vi "Get or Add TableDefinitionPart.vi"(7 "Sheet Name":string, 8 "error in":errorcluster, 10 "Table Name":string, 11 "SpreadsheetDoc in":refnum<k24>) -> (0 "error out":errorcluster, 2 "TableDefinitionPart":refnum<k24>, 3 "SpreadsheetDo out":refnum<k24>, 5 "Sheet Name":string)   [LabVIEW 2019, in "Open Xml.lvlib"]
uses:
  Open Xml.lvlib
  D:/git/Open-Xml-LabVIEW/Source/OpenXmlGenericsWrapper.dll
  OpenXmlGenericsWrapper.dll
  D:/git/Open-Xml-LabVIEW/Source/DocumentFormat.OpenXml.dll
  DocumentFormat.OpenXml.dll
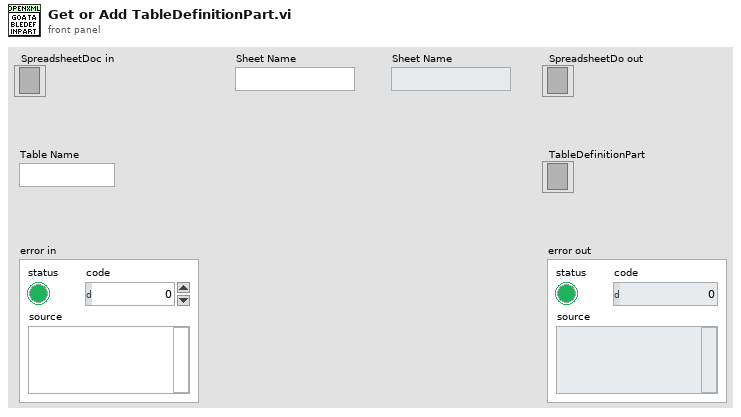
[diagram p1: front panel]
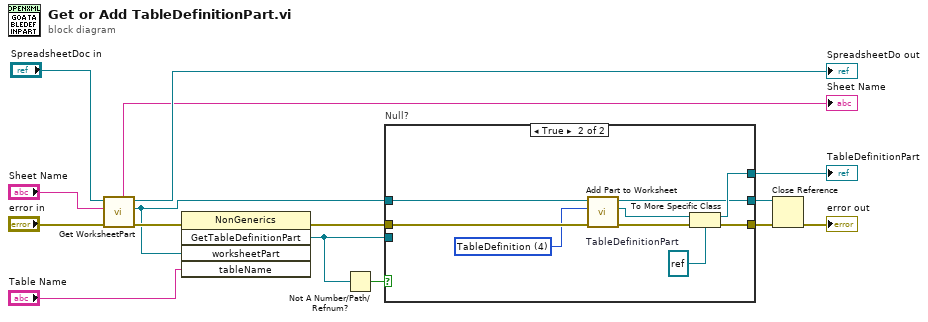
[diagram p0: block diagram]
diagram:
  n1 = call "Get WorksheetPart.vi"("error in"="error in", "Sheet Name"="Sheet Name", "SpreadsheetDoc in"="SpreadsheetDoc in") -> ("error out"=w12:errorcluster, "WorksheetPart"=w1:refnum<k24>, "SpreadsheetDoc out"=→"SpreadsheetDo out":refnum<k24>, "SheetName"=→"Sheet Name":string)  [unwired: 5 in]
  n2 = invoke class="NonGenerics" method="GetTableDefinitionPart"(error in=w12, "worksheetPart"=w1, "tableName"="Table Name") -> (error out=w5:errorcluster, "GetTableDefinitionPart"=w7:refnum<k24>)  [unwired: 2 in, 3 out]
  n3 = Not A Number/Path/Refnum?(number/path/refnum=w7) -> (NaN/Path/Refnum?=w8:bool)
  n4 = case "Null?" shown="True" w8 {
    tunnel: w7 -> [w18 _]
    tunnel: w5 -> [w17 w27]
    tunnel: [w17 w25] -> w2
    tunnel: [w18 w23] -> w6
    tunnel: w1 -> [w16 w22]
    tunnel: [w16 w19] -> w3
    frame False {
    }
    frame True {
      w21 = 4 items=["Chart", "Drawings", "ImagePart", "PivotTable", "TableDefinition", "WorksheetComments", "WorksheetDrawing"] ("PartType")
      w24 = refnum<k24> refnum  # TableDefinitionPart
      n5 = call "Add Part to Worksheet.vi"("error in"=w27, "PartType"=w21, "WorksheetPart in"=w22) -> ("error out"=w26:errorcluster, "Open Xml Part"=w20:refnum<k24>, "WorksheetPart out"=w19:refnum<k24>)  [unwired: 6 in]
      n6 = To More Specific Class(target class=w24, reference=w20, error in=w26) -> (specific class reference=w23:refnum<k24>, error out=w25:errorcluster)
    }
  }
  "TableDefinitionPart" <- w6
  n7 = Close Reference(reference=w3, error in (no error)=w2) -> (error out=→"error out":errorcluster)
